vi "BK Precision 9200 Series Output DC Volts.vi"() -> ()   [LabVIEW 2021]
doc: "This example shows how to configure the instrument's output voltage level and over voltage protection. The actual voltage level and actual current level are returned."
uses:
  <instrlib>/BK Precision 9200 Series/BK Precision 9200 Series.lvlib
panel:
  in  "Current Limit (1.0 A)":dbl=1.0 format="%.3g"
  in  "Enable OVP (T: Enable)":bool=TRUE
  in  "Stop Output":bool
  in  "Voltage Limit (66V)":dbl=66.0 format="%.2f"
  out "Actual Current Limit (A)":dbl format="%.3f"
  out "Actual Voltage Level (V)":dbl format="%.3f"
  in  "Voltage Level (1.0 V)":dbl=1.0 format="%.3f"
  in  "VISA resource name":refnum<visa-resource-name>
  # "(c) 2014 B&K Precision Corporation.  ALL RIGHTS RESERVED."
  # "Over Voltage Protection"
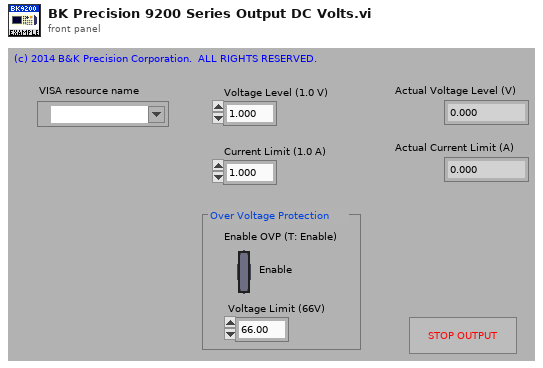
[diagram p1: front panel]
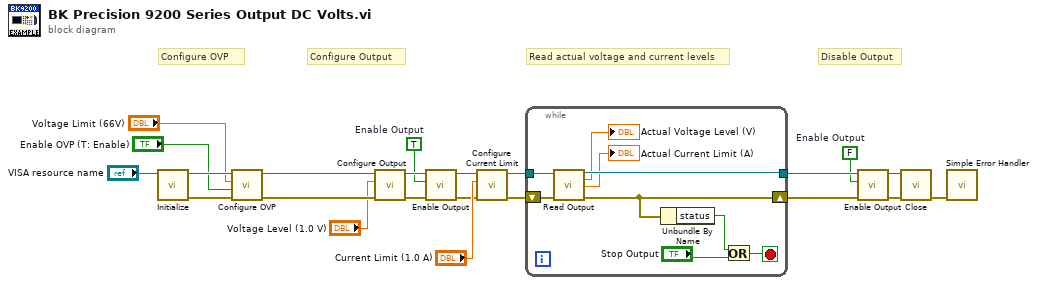
[diagram p0: block diagram]
diagram:
  w6 = FALSE  # Enable Output
  w1 = TRUE  # Enable Output
  # "Disable Output"
  # "Read actual voltage and current levels"
  # "Configure Output"
  # "Configure OVP"
  n1 = call <instrlib>:"Initialize.vi"("VISA resource name"="VISA resource name") -> ("error out"=w20:errorcluster, "VISA resource name out"=w19:refnum<visa-resource-name>)  [unwired: 9 in]
  n2 = call <instrlib>:"Configure OVP.vi"("error in (no error)"=w20, "Enable OVP (T: Enable)"="Enable OVP (T: Enable)", "Voltage Limit (66.000 V)"="Voltage Limit (66V)", "VISA resource name"=w19) -> ("error out"=w16:errorcluster, "VISA resource name out"=w17:refnum<visa-resource-name>)  [unwired: 6 in]
  n3 = call <instrlib>:"Configure Output.vi"("error in (no error)"=w16, "Voltage Level (0.0 V)"="Voltage Level (1.0 V)", "VISA resource name"=w17) -> ("error out"=w4:errorcluster, "VISA resource name out"=w5:refnum<visa-resource-name>)  [unwired: 7 in]
  n4 = call <instrlib>:"Enable Output.vi"("error in (no error)"=w4, "Enable Output (F: False)"=w1, "VISA resource name"=w5) -> ("error out"=w3:errorcluster, "VISA resource name out"=w2:refnum<visa-resource-name>)  [unwired: 7 in]
  n5 = call <instrlib>:"Configure Current Limit.vi"("error in (no error)"=w3, "Current Limit (0.0 A)"="Current Limit (1.0 A)", "VISA resource name"=w2) -> ("error out"=w12:errorcluster, "VISA resource name out"=w11:refnum<visa-resource-name>)  [unwired: 7 in]
  n6 = while {
    tunnel: w11 -> [w28]
    tunnel: [w25] -> w15
    shift-right: [w26] -> w7
    shift-left: w12 -> [w27]
    stop <- w31 stop-if-true
    n7 = call <instrlib>:"Read Output.vi"("VISA resource name"=w28, "error in (no error)"=w27) -> ("VISA resource name out"=w25:refnum<visa-resource-name>, "Actual Voltage Level (V)"=→"Actual Voltage Level (V)":dbl, "Actual Current Level (A)"=→"Actual Current Limit (A)":dbl, "error out"=w26:errorcluster)  [unwired: 9 in, 1 out]
    n8 = Unbundle By Name(w26) -> ("status"=w29:bool)
    n9 = Or(x=w29, y="Stop Output") -> (x .or. y?=w31:bool)
  }
  n10 = call <instrlib>:"Enable Output.vi"("error in (no error)"=w7, "Enable Output (F: False)"=w6, "VISA resource name"=w15) -> ("error out"=w13:errorcluster, "VISA resource name out"=w14:refnum<visa-resource-name>)  [unwired: 7 in]
  n11 = call <instrlib>:"Close.vi"("error in (no error)"=w13, "VISA resource name"=w14) -> ("error out"=w21:errorcluster)  [unwired: 9 in]
  n12 = call <vilib>:"Simple Error Handler.vi"("error in (no error)"=w21) -> ()  [unwired: 4 in, 5 out]
